vi "Read lvlibretls server listener.vi"(8 "error in":errorcluster, 11 "TLS HTTP server in":refnum<class "TLS HTTP server.lvclass">) -> (0 "error out":errorcluster, 2 "lvlibretls server listener":refnum<class "lvlibretls server listener.lvclass">, 3 "TLS HTTP server out":refnum<class "TLS HTTP server.lvclass">)   [LabVIEW 2016, in "TLS HTTP server.lvclass"]
uses:
  TLS HTTP server.lvclass
  lvlibtls/server/lvlibretls server listener.lvclass
  TLS HTTP server.lvclass/TLS HTTP server.ctl
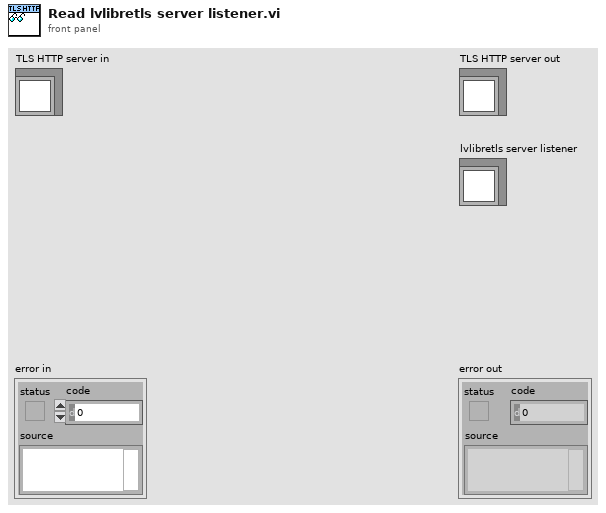
[diagram p1: front panel]
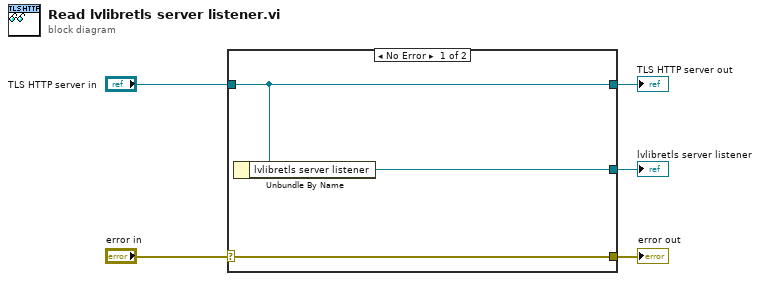
[diagram p0: block diagram]
diagram:
  n1 = case shown="No Error" "error in" {
    selector: "error in" -> [w8 w9]
    tunnel: [w8 w9] -> w4
    tunnel: [w7 w10] -> w2
    tunnel: "TLS HTTP server in" -> [w7 w10]
    tunnel: [w6 _] -> w1
    frame No Error {
      n2 = Unbundle By Name(w7) -> ("lvlibretls server listener"=w6:refnum<class "lvlibretls server listener.lvclass">)
    }
    frame Error {
    }
  }
  "error out" <- w4
  "TLS HTTP server out" <- w2
  "lvlibretls server listener" <- w1
